vi "dvp Vi Set Quick Roi Sel.vi"(10 "QuickRoiSel":u32, 11 "handle":u32) -> (3 "function return":u32(ring))   [LabVIEW 2018, in "LabViewDVPCamera.lvlib"]
doc: "LabviewDvp2Api dvpStatus dvpViSetQuickRoiSel(dvpHandle handle, dvpUint32 QuickRoiSel);"
uses:
  LabViewDVPCamera.lvlib
  LabViewDVPCamera/LabViewDVPCamera.dll
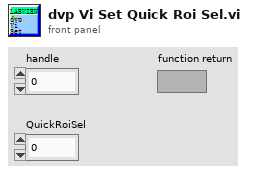
[diagram p1: front panel]
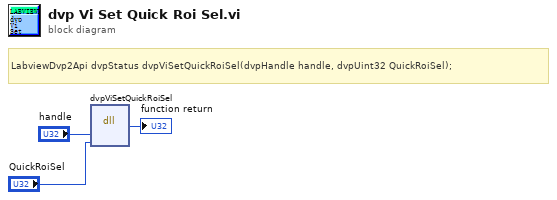
[diagram p0: block diagram]
diagram:
  # "LabviewDvp2Api dvpStatus dvpViSetQuickRoiSel(dvpHandle handle, dvpUint32 QuickRoiSel);"
  n1 = dll-call lib="C:/Program Files (x86)/DVP2 Labview cn 64/Sample/LabViewDVPCamera/LabViewDVPCamera.*" fn="dvpViSetQuickRoiSel"("handle"="handle", "QuickRoiSel"="QuickRoiSel") -> (→"function return":u32)  [unwired: 5 in, 2 out]
